vi "Burst Apply.vi"(8 "error in (no error)":errorcluster, 9 "Waveform in":dbl[](array[numeric]), 10 "Sampling Rate (Hz)":dbl, 11 "Burst":T1) -> (0 "error out":errorcluster, 1 "Gated waveform":dbl[](array[numeric]))   [LabVIEW 2020]
uses:
  Controls/Burst XCtl/Burst Data.ctl
  Controls/Burst XCtl/Burst Control.xctl
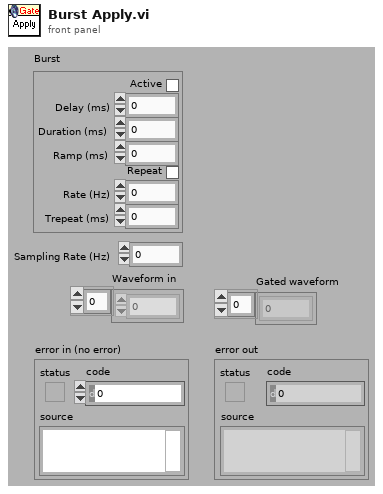
[diagram p1: front panel]
types:
  T1 = typedef "Burst Control.xctl/Burst Data.ctl" = cluster{"Active":bool, "Delay (ms)":dbl, "Duration (ms)":dbl, "Ramp (ms)":dbl, "Rate (Hz)":dbl, "Trepeat (ms)":dbl, "Repeat":bool}
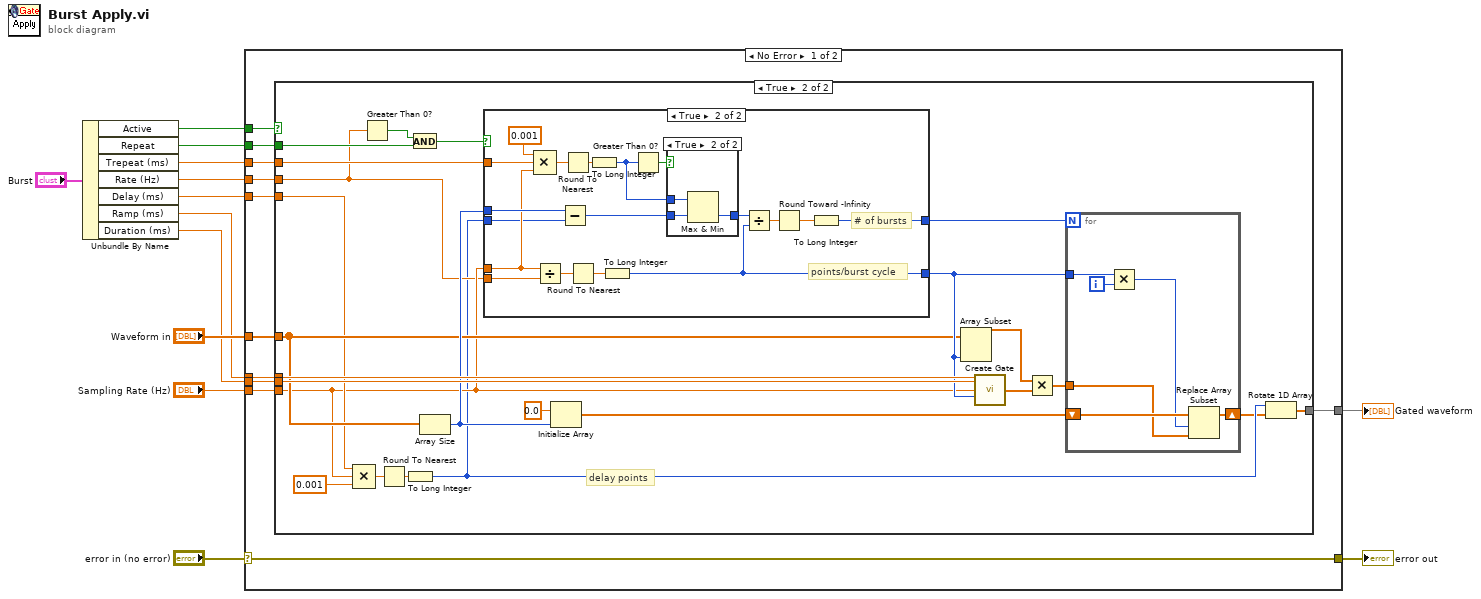
[diagram p0: block diagram]
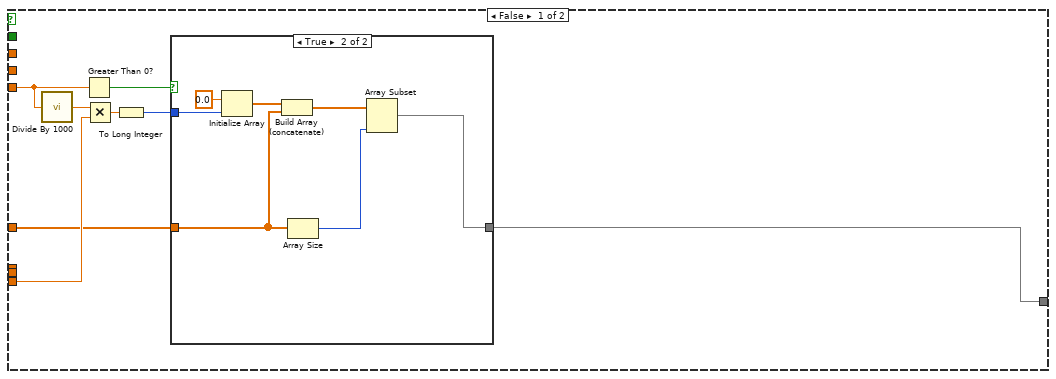
[diagram p2: hidden frame]
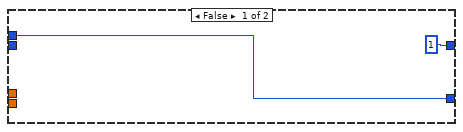
[diagram p4: hidden frame]
diagram:
  n1 = Unbundle By Name("Burst") -> ("Active"=w11:bool, "Repeat"=w8:bool, "Trepeat (ms)"=w7:dbl, "Rate (Hz)"=w3:dbl, "Delay (ms)"=w1:dbl, "Ramp (ms)"=w5:dbl, "Duration (ms)"=w4:dbl)
  n2 = case shown="No Error" "error in (no error)" {
    selector: "error in (no error)" -> [w19 w95]
    tunnel: w11 -> [w14 _]
    tunnel: "Waveform in" -> [w21 _]
    tunnel: [w19 w95] -> w9
    tunnel: w5 -> [w23 _]
    tunnel: w4 -> [w22 _]
    tunnel: w8 -> [w24 _]
    tunnel: "Sampling Rate (Hz)" -> [w16 _]
    tunnel: w7 -> [w15 _]
    tunnel: [w20 _] -> w6
    tunnel: w3 -> [w18 _]
    tunnel: w1 -> [w17 _]
    frame No Error {
      n3 = case shown="True" w14 {
        tunnel: w24 -> [_ w49]
        tunnel: w23 -> [_ w64]
        tunnel: w22 -> [_ w63]
        tunnel: w15 -> [_ w50]
        tunnel: w21 -> [w28 w56]
        tunnel: [w25 w46] -> w20
        tunnel: w18 -> [_ w48]
        tunnel: w17 -> [w32 w55]
        tunnel: w16 -> [w30 w54]
        frame False {
          n4 = call "Divide By 1000.vi"("X"=w32) -> ("X/1000"=w31:dbl)
          n5 = Greater Than 0?(x=w32) -> (x > 0?=w27:bool)
          n6 = Multiply(x=w31, y=w30) -> (x*y=w29:dbl)
          n7 = To Long Integer(number=w29) -> (32bit integer=w26:i32)
          n8 = case shown="True" w27 {
            tunnel: w28 -> [w33 w36]
            tunnel: w26 -> [_ w40]
            tunnel: [w33 w34] -> w25
            frame False {
            }
            frame True {
              n9 = Initialize Array(0.0 ("element"), w40) -> (w38:dbl[])
              n10 = Build Array (concatenate)(w38, w36) -> (w37:dbl[])
              n11 = Array Size(array=w36) -> (size(s)=w35:i32)
              n12 = Array Subset(array=w37, length=w35) -> (w34:dbl[])  [unwired: 1 in]
            }
          }
        }
        frame True {
          # "delay points"
          n13 = Compound Arithmetic op=MULTIPLY(w55, w54, 0.001 ("value")) -> (w52:dbl)
          n14 = Greater Than 0?(x=w48) -> (x > 0?=w51:bool)
          n15 = Round To Nearest(number=w52) -> (nearest integer value=w53:dbl)
          n16 = To Long Integer(number=w53) -> (32bit integer=w44:i32)
          n17 = And(x=w51, y=w49) -> (x .and. y?=w47:bool)
          n18 = Array Size(array=w56) -> (size(s)=w62:i32)
          n19 = case shown="True" w47 {
            tunnel: w62 -> [w72 w85]
            tunnel: w54 -> [_ w78]
            tunnel: [w72 w83] -> w57
            tunnel: w50 -> [_ w88]
            tunnel: [1 w80] -> w60
            tunnel: w48 -> [_ w77]
            tunnel: w44 -> [_ w75]
            frame False {
            }
            frame True {
              # "# of bursts"
              # "points/burst cycle"
              n20 = Compound Arithmetic op=MULTIPLY(0.001 ("value"), w88, w78) -> (w87:dbl)
              n21 = Divide(x=w78, y=w77) -> (x/y=w90:dbl)
              n22 = Subtract(x=w85, y=w75) -> (x-y=w76:i32)
              n23 = Round To Nearest(number=w87) -> (nearest integer value=w86:dbl)
              n24 = Round To Nearest(number=w90) -> (nearest integer value=w89:dbl)
              n25 = To Long Integer(number=w86) -> (32bit integer=w74:i32)
              n26 = To Long Integer(number=w89) -> (32bit integer=w83:i32)
              n27 = Greater Than 0?(x=w74) -> (x > 0?=w73:bool)
              n28 = case shown="True" w73 {
                tunnel: w74 -> [_ w94]
                tunnel: [w91 w93] -> w84
                tunnel: w76 -> [w91 w92]
                frame False {
                }
                frame True {
                  n29 = Max & Min(x=w94, y=w92) -> (min(x,y)=w93:i32)  [unwired: 1 out]
                }
              }
              n30 = Divide(x=w84, y=w83) -> (x/y=w82:dbl)
              n31 = Round Toward -Infinity(1:w82) -> (0:w81:dbl)
              n32 = To Long Integer(number=w81) -> (32bit integer=w80:i32)
            }
          }
          n33 = Initialize Array(0.0 ("element"), w62) -> (w58:dbl[])
          n34 = Array Subset(array=w56, length=w57) -> (w42:dbl[])  [unwired: 1 in]
          n35 = call "Create Gate.vi"("Ramp (ms)"=w64, "Duration (ms)"=w63, "Sampling Rate (Hz)"=w54, "Npts"=w57) -> ("Gate"=w59:dbl[])  [unwired: 10 in, 1 out]
          n36 = Multiply(x=w42, y=w59) -> (x*y=w43:dbl[])
          n37 = for {
            N: w60 -> [_]
            tunnel: w43 -> [w68]
            shift-right: [w69] -> w41
            shift-left: w58 -> [w70]
            tunnel: w57 -> [w66]
            i -> [w67]
            n38 = Multiply(x=w66, y=w67) -> (x*y=w65:i32)
            n39 = Replace Array Subset(array=w70, new element=w68, index=w65) -> (w69:dbl[])
          }
          n40 = Rotate 1D Array(1:w41, 2:w44) -> (0:w46:dbl[])
        }
      }
    }
    frame Error {
    }
  }
  "error out" <- w9
  "Gated waveform" <- w6
